vi "Send Internal Stop.vi"(8 "Error in":errorcluster, 11 "Queue Data":T1) -> (0 "Error out":errorcluster)   [LabVIEW 2018, in "Event Messaging.lvlib"]
uses:
  Event Messaging.lvlib
  QMH Template/Type Defs/EventsAndQueues--cluster.ctl
  Queue Messaging/Type Defs/Queue Message--cluster.ctl
  Type Defs/Event Message--cluster.ctl
  Queue Messaging/Queue Messaging.lvlib
  QMH/QMH CORE.lvlib
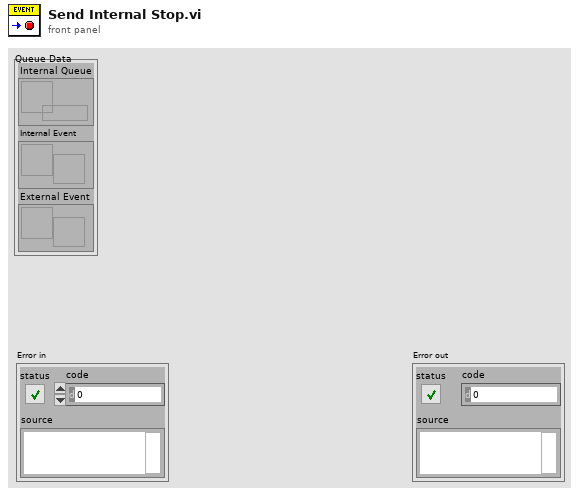
[diagram p1: front panel]
types:
  T1 = typedef "QMH CORE.lvlib/EventsAndQueues--cluster.ctl" = cluster{"Internal Queue":refnum<queue>, "Internal Event":refnum<user-event>, "External Event":refnum<user-event>}
  T2 = typedef "Event Messaging.lvlib/Event Message--cluster.ctl" = cluster{"Cmd":string, "Data":variant}
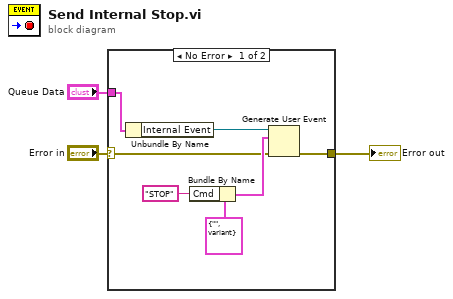
[diagram p0: block diagram]
diagram:
  n1 = case shown="No Error" "Error in" {
    selector: "Error in" -> [w6 w11]
    tunnel: [w5 w11] -> w2
    tunnel: "Queue Data" -> [w4 _]
    frame No Error {
      n2 = Unbundle By Name(w4) -> ("Internal Event"=w10:refnum<user-event>)
      n3 = Bundle By Name(cluster=T2 {"Cmd"="", "Data"=variant} ("event data"), "Cmd"="STOP") -> (w8:T2)
      n4 = Generate User Event(user event=w10, event data cluster=w8, error in=w6) -> (error out=w5:errorcluster)  [unwired: 1 in, 1 out]
    }
    frame Error {
    }
  }
  "Error out" <- w2
